vi "Taiko_Demo_WndMsg.vi"() -> ()   [LabVIEW 2010]
uses:
  Types/Taiko_Cmds.ctl
  Types/Taiko_Data.ctl
  _lib/PDLM/pdlm_lib_x86_x64_UIThread.llb/PDLM_Tag.ctl
  _lib/PDLM/pdlm_lib_x86_x64_UIThread.llb/PDLM_TaggedValue.ctl
  _lib/PDLM/pdlm_lib_x86_x64_UIThread.llb/PDLM_TaggedValueList.ctl
  <vilib>/Utility/miscctls.llb/LVRowAndColumnTypeDef.ctl
  _lib/Windows Messages for Labview/Windows messages for Labview (32 and 64).lvlib
  Types/ScaleDisplayParams.ctl
  Types/ControlAttributes.ctl
  _lib/PDLM/pdlm_lib_x86_x64_UIThread.llb/PDLM_TriggerMode.ctl
  SubVIs/AddControlsToControlStateArray.vi
  _lib/PDLM/pdlm_lib_x86_x64_UIThread.llb/PDLM_PulseTableIDs.ctl
  Types/selector.ctl
panel:
  out "Info":string="Library Version:\n1.0.64.3114\n\nSerials:\n1234567\r\n"
  in  "SetSelector":T1 caption="Select:"
  in  "LDH Pulse Table IDs":T2
  in  "Slide":sgl(slide) min=0 max=100 step=0.1 scale=0.0..100.0
  out "Tagged Value List":i32[](listbox)
  out "SystemStatus":i32(listbox)=-1
  out "SystemStatusText":string="queued error message pending\nlocked by key lock\nlocked by on/off button\nparameter changes pending\nexclusive software operation granted"
  out "QError":string="queued error message pending\nlocked by key lock\nlocked by on/off button\nparameter changes pending\nexclusive software operation granted"
  out "LH Info & Data":i32(listbox)=-1
  out "LHFeatures":i32(listbox)=-1
  out "LHFeaturesText":string="pulse mode option (int. & ext. triggerable)\ncontinuous-wave option\nburst mode option (int. triggerable)\nfan-cooled (switchable)\nintensity sensor option (type=1)"
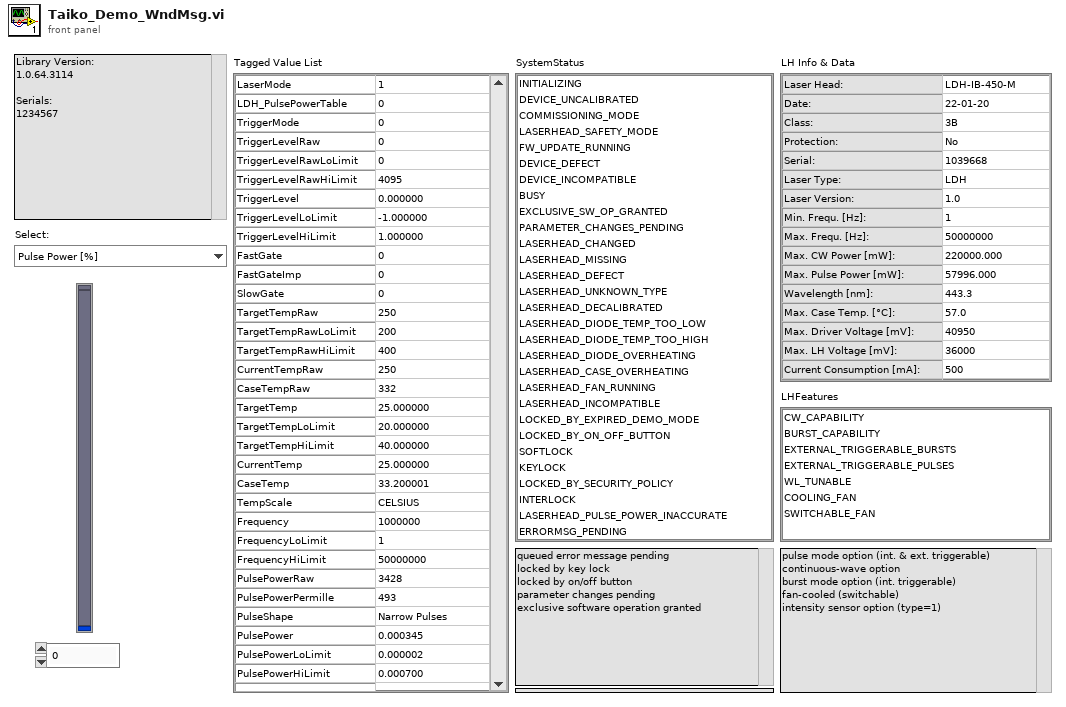
[diagram p1: front panel]
types:
  T1 = typedef "selector.ctl" = enum16{"Pulse Power [%]", "Frequency [Hz]", "Trigger Level [V]", "Pulse Table"}
  T2 = typedef "PDLM_PulseTableIDs.ctl" = enum16{"LDH_LIN_PULSE_POWER_TABLE", "LDH_MAX_PULSE_POWER_TABLE"}
  T3 = typedef "Taiko_Data.ctl" = cluster{"USBIdx":i32, "Error":errorcluster, "TaggedValueList":T4, "Ctrl State Arr":T7[], "Scale Display Params":T8}
  T4 = typedef "PDLM_TaggedValueList.ctl" = T5[]
  T5 = typedef "PDLM_TaggedValue.ctl" = cluster{"Tag":T6, "Value":u32}
  T6 = typedef "PDLM_Tag.ctl" = u32
  T7 = typedef "ControlAttributes.ctl" = cluster{"Ctl Refnum":refnum<vi>, "Visible":bool, "Enabled state":enum8{"Enabled", "Disabled", "Disabled and Grayed Out"}}
  T8 = typedef "ScaleDisplayParams.ctl" = cluster{"Style":u8, "MapMode":u8, "Increment":dbl, "Minimum":dbl, "Maximum":dbl, "Value":dbl}
  T9 = typedef "Taiko_Cmds.ctl" = enum16{"Idle", "Init", "Exit", "Update", "Error"}
  T10 = typedef "Windows messages for Labview (32 and 64).lvlib/Win Msg Queue RefNum.ctl" = refnum<k1>
  T11 = typedef "PDLM_TriggerMode.ctl" = enum32{"INTERNAL", "EXTERNAL_FALLING_EDGE", "EXTERNAL_RISING_EDGE"}
  T12 = typedef "LVRowAndColumnTypeDef.ctl" = cluster{"Row":i32, "Column":i32}
  T13 = enum16{"Pulse Power [%]", "Frequency [Hz]", "Trigger Level [V]"}
  T14 = typedef "Windows messages for Labview (32 and 64).lvlib/windows message x64.ctl" = cluster{"hWnd":u64, "Msg":u32, "wParam":u64, "lParam":i32, "time":u32, "point":cluster{"X":i32, "Y":i32}}
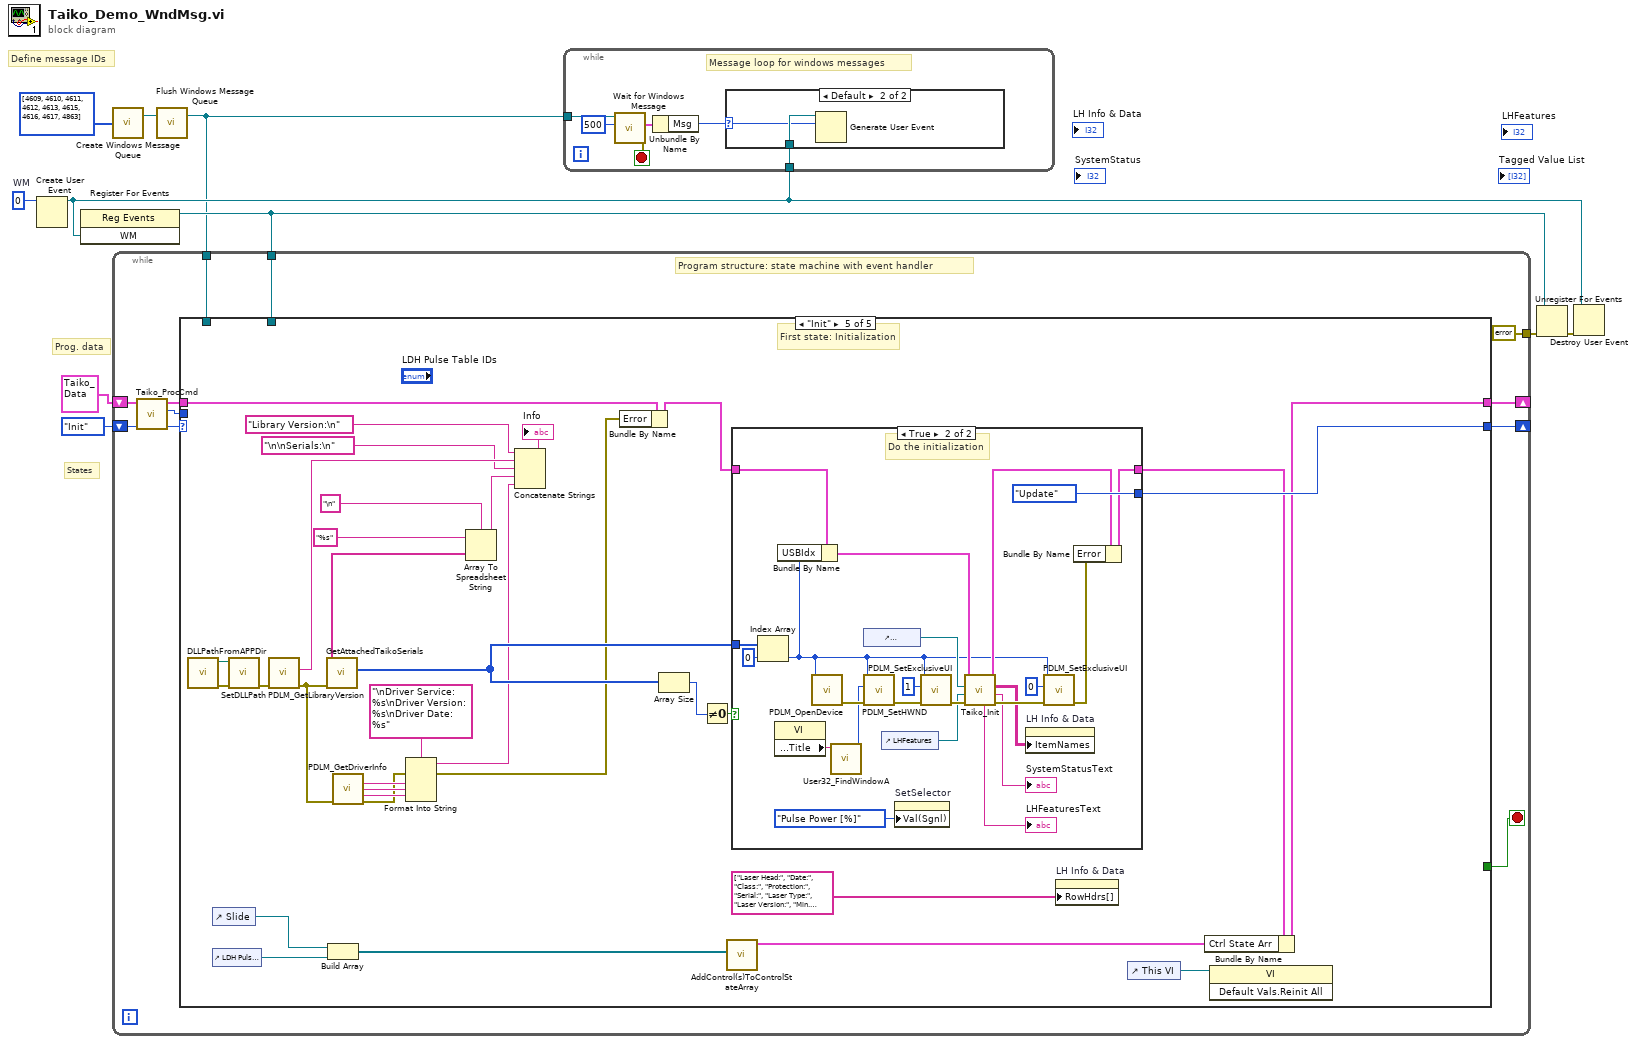
[diagram p0: block diagram]
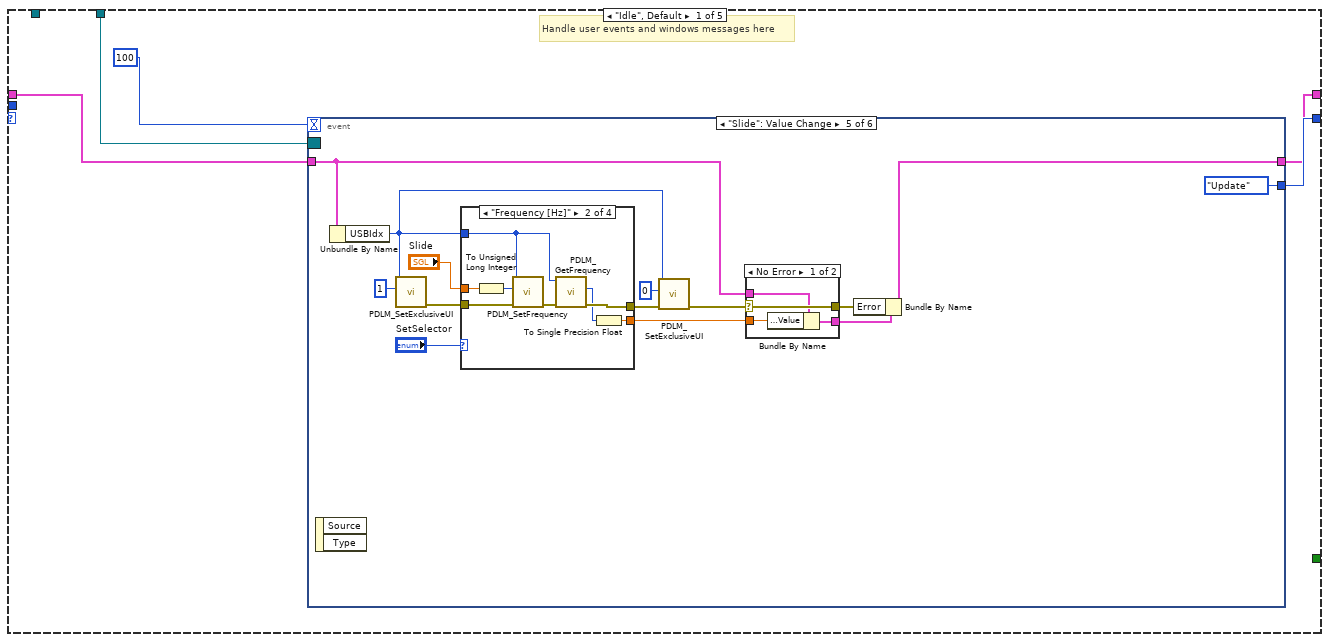
[diagram p3: hidden frame]
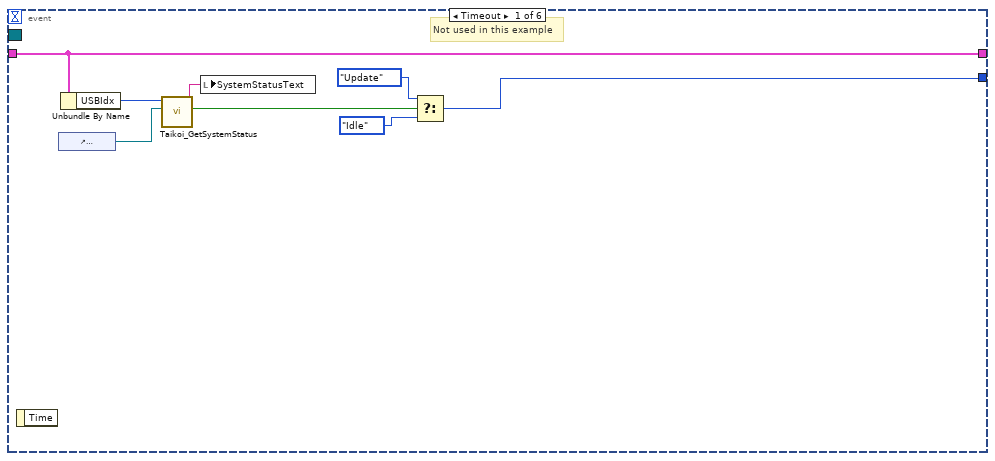
[diagram p4: hidden frame]
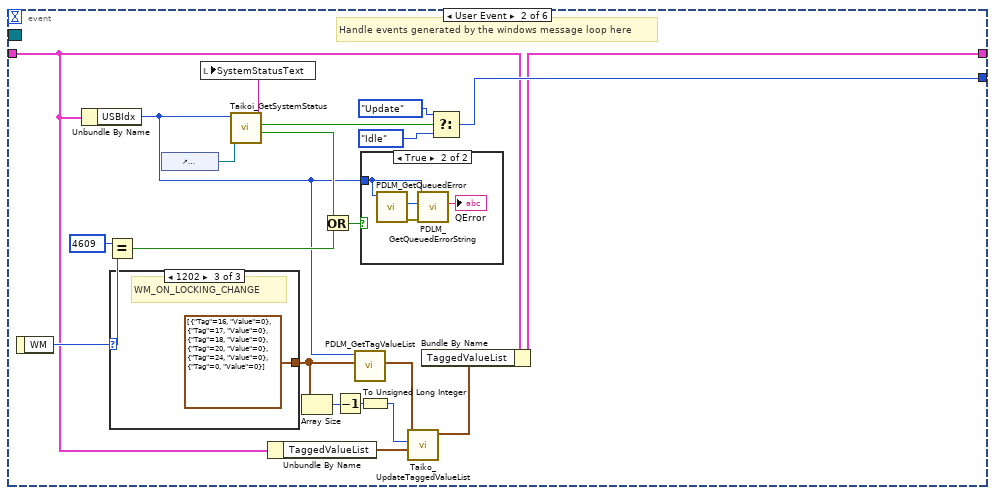
[diagram p5: hidden frame]
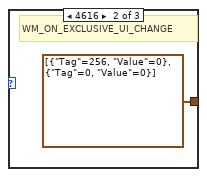
[diagram p7: hidden frame]
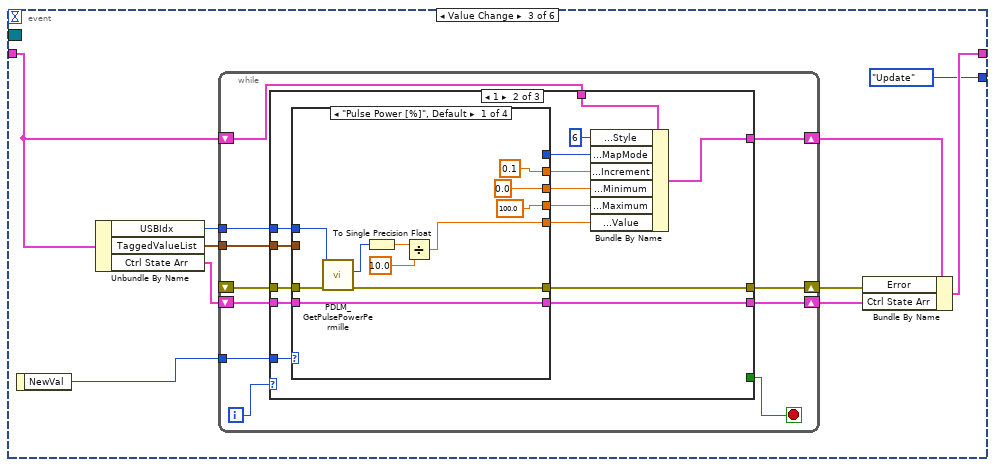
[diagram p9: hidden frame]
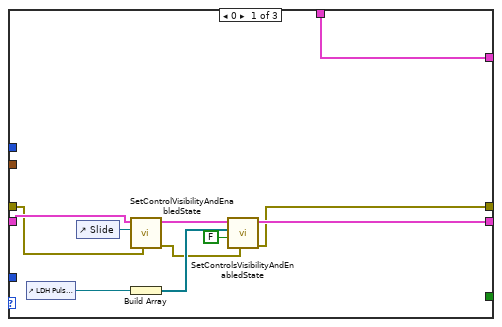
[diagram p10: hidden frame]
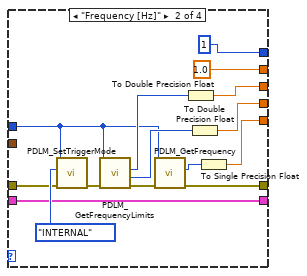
[diagram p11: hidden frame]
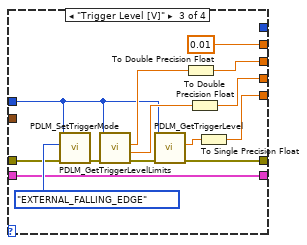
[diagram p12: hidden frame]
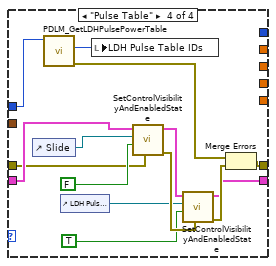
[diagram p13: hidden frame]
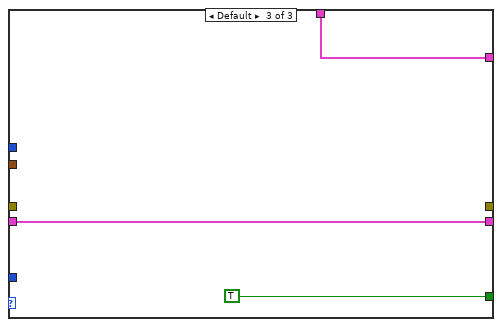
[diagram p14: hidden frame]
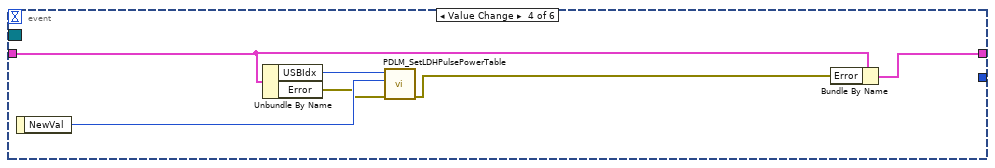
[diagram p15: hidden frame]
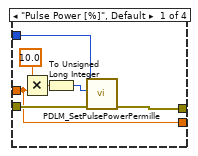
[diagram p17: hidden frame]
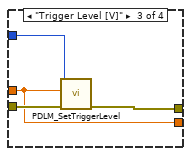
[diagram p18: hidden frame]
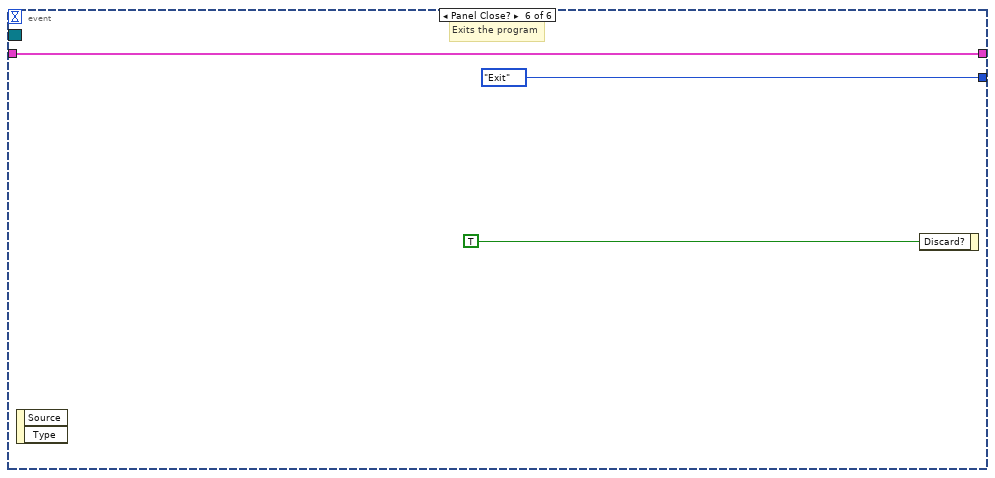
[diagram p20: hidden frame]
diagram:
  w1 = u32 0  # WM
  # "Prog. data"
  # "States"
  # "Define message IDs"
  n1 = Create User Event(user event datatype=w1) -> (user event=w3:refnum<user-event>)  [unwired: 1 in, 1 out]
  n2 = register-events(w3) -> (reference out=w6:refnum<event-registration>)  [unwired: 2 in, 1 out]
  n3 = call "Create Windows Message Queue.vi"("Messeges (none)"=u32[] [4609, 4610, 4611, 4612, 4613, 4615, 4616, 4617, 4863]) -> ("win msg queue"=w7:T10)  [unwired: 2 in, 1 out]
  n4 = call "Flush Windows Message Queue.vi"("win msg queue"=w7) -> ("win msg queue out"=w2:T10)  [unwired: 1 in, 1 out]
  n5 = while {
    shift-right: [w20] -> _
    shift-left: Taiko_Cmds."Init" ("Cmd") -> [w16]
    shift-right: [w19] -> _
    shift-left: T3 {"USBIdx"=0, "Error"={"status"=FALSE, "code"=0, "source"=""}, "TaggedValueList"=[], "Ctrl State Arr"=[], "Scale Display Params"={"Style"=0, "MapMode"=0, "Increment"=0.0, "Minimum"=0.0, "Maximum"=0.0, "Value"=0.0}} ("Data") -> [w18]
    tunnel: w6 -> [w14]
    tunnel: [errorcluster {"status"=FALSE, "code"=0, "source"=""} ("error constant")] -> w4
    tunnel: w2 -> [w12]
    stop <- w21 stop-if-true
    # "Program structure: state machine with event handler"
    n6 = call "Taiko_ProcCmd.vi"("Cmd in"=w16, "Data in"=w18) -> ("Cmd out"=w15:T9, "Cmd prev"=w11:T9, "Data out"=w17:T3)  [unwired: 7 in]
    n7 = case shown="\"Init\"" w15 {
      tunnel: [_ TRUE _ _ _] -> w21
      tunnel: [w25 _ w221 _ w296] -> w20
      tunnel: w17 -> [w23 w218 w226 w241 w295]
      tunnel: [w24 w218 w225 w249 w273] -> w19
      tunnel: w14 -> [w22 _ _ _ _]
      tunnel: w12 -> [_ w215 _ _ _]
      tunnel: w11 -> [_ _ w220 _ _]
      frame "Idle", Default {
        # "Handle user events and windows messages here"
        n8 = event shown="[4] \"Slide\": Value Change" {
          selector: w22 -> [_ _ _ _ _ _]
          dyn-events: _ -> [_ _ _ _ _ _]
          timeout: 100 -> [_ _ _ _ _ _]
          tunnel: [w29 w52 Taiko_Cmds."Update" ("Cmd") _ Taiko_Cmds."Update" ("Cmd") Taiko_Cmds."Exit" ("Cmd")] -> w25
          tunnel: [w33 w40 w63 w168 w183 w212] -> w24
          tunnel: w23 -> [w33 w41 w67 w169 w176 w212]
          event Timeout {
            # "Not used in this example"
            n9 = event-data() -> ()  [unwired: 1 in, 1 out]
            n10 = control-ref of="SystemStatus"() -> (w34:refnum<vi>)
            n11 = Unbundle By Name(w33) -> ("USBIdx"=w32:i32)
            n12 = call "Taikoi_GetSystemStatus.vi"("LBSysStatRef"=w34, "USBIdx"=w32) -> ("needUpdate"=w27:bool, "Status"=w28:string)  [unwired: 6 in, 2 out]
            n13 = local write "SystemStatusText"(w28) -> ()
            n14 = Select(t=Taiko_Cmds."Update" ("Cmd"), s=w27, f=Taiko_Cmds."Idle") -> (s? t:f=w29:T9)
          }
          event User Event {
            # "Handle events generated by the windows message loop here"
            n15 = event-data() -> ("WM"=w49:u32)  [unwired: 1 in]
            n16 = Unbundle By Name(w41) -> ("USBIdx"=w35:i32)
            n17 = Equal?(x=u32 4609, y=w49) -> (x = y?=w47:bool)
            n18 = case shown="1202" w49 {
              tunnel: [_ T4 [{"Tag"=256, "Value"=0}, {"Tag"=0, "Value"=0}] ("TaggedValueList") T4 [{"Tag"=16, "Value"=0}, {"Tag"=17, "Value"=0}, {"Tag"=18, "Value"=0}, {"Tag"=20, "Value"=0}, {"Tag"=24, "Value"=0}, {"Tag"=0, "Value"=0}] ("TaggedValueList")] -> w39
              frame 0, Default {
              }
              frame 4616 {
                # "WM_ON_EXCLUSIVE_UI_CHANGE"
              }
              frame 4610 {
                # "WM_ON_LOCKING_CHANGE"
              }
            }
            n19 = control-ref of="SystemStatus"() -> (w55:refnum<vi>)
            n20 = call "Taikoi_GetSystemStatus.vi"("LBSysStatRef"=w55, "USBIdx"=w35) -> ("QError"=w46:bool, "needUpdate"=w50:bool, "Status"=w51:string)  [unwired: 6 in, 1 out]
            n21 = local write "SystemStatusText"(w51) -> ()
            n22 = Unbundle By Name(w41) -> ("TaggedValueList"=w42:T4)
            n23 = Array Size(array=w39) -> (size(s)=w38:i32)
            n24 = Or(x=w46, y=w47) -> (x .or. y?=w45:bool)
            n25 = Decrement(x=w38) -> (x-1=w37:i32)
            n26 = call "PDLM_GetTagValueList.vi"("TaggedValueList"=w39, "USBIdx"=w35) -> ("TaggedValueList out"=w44:T4)  [unwired: 7 in, 2 out]
            n27 = To Unsigned Long Integer(number=w37) -> (unsigned 32bit integer=w36:u32)
            n28 = case shown="True" w45 {
              tunnel: w35 -> [_ w59]
              frame False {
              }
              frame True {
                n29 = call "PDLM_GetQueuedError.vi"("USBIdx"=w59) -> ("error out"=w61:errorcluster, "ErrCode"=w60:i32)  [unwired: 8 in, 1 out]
                n30 = call "PDLM_GetQueuedErrorString.vi"("error in (no error)"=w61, "ErrCode"=w60, "USBIdx"=w59) -> ("ErrText"=→"QError":string)  [unwired: 6 in, 2 out]
              }
            }
            n31 = call "Taiko_UpdateTaggedValueList.vi"("TaggedValueList all"=w42, "ListLen in"=w36, "TaggedValueList in"=w44) -> ("TaggedValueList"=w43:T4)  [unwired: 7 in, 1 out]
            n32 = Bundle By Name(cluster=w41, "TaggedValueList"=w43) -> (w40:T3)
            n33 = Select(t=Taiko_Cmds."Update" ("Cmd"), s=w50, f=Taiko_Cmds."Idle") -> (s? t:f=w52:T9)
          }
          event Value Change {
            n34 = event-data() -> ("NewVal"=w68:T1)  [unwired: 1 in]
            n35 = Unbundle By Name(w67) -> ("USBIdx"=w69:i32, "TaggedValueList"=w70:T4, "Ctrl State Arr"=w71:T7[])
            n36 = while {
              tunnel: w69 -> [w82]
              tunnel: w68 -> [w81]
              tunnel: w70 -> [w79]
              shift-right: [w78] -> w66
              shift-left: w71 -> [w77]
              shift-right: [w80] -> w65
              shift-left: _ -> [w74]
              shift-right: [w72] -> w64
              shift-left: w67 -> [w73]
              i -> [w76]
              stop <- w75 stop-if-true
              n37 = case shown="1" w76 {
                tunnel: w82 -> [_ w108 _]
                tunnel: w81 -> [_ w107 _]
                tunnel: [w84 w106 _] -> w80
                tunnel: w79 -> [_ w105 _]
                tunnel: [w88 w103 w164] -> w78
                tunnel: w77 -> [w90 w104 w164]
                tunnel: [_ _ TRUE] -> w75
                tunnel: w74 -> [w83 w102 _]
                tunnel: w73 -> [w87 w101 w163]
                tunnel: [w87 w100 w163] -> w72
                frame 0 {
                  n38 = control-ref of="LDH Pulse Table IDs"() -> (w86:refnum<vi>)
                  n39 = control-ref of="Slide"() -> (w92:refnum<vi>)
                  n40 = call "SetControlVisibilityAndEnabledState.vi"("error in (no error)"=w83, "Ctl Refnum"=w92, "Control State Array"=w90) -> ("error out"=w85:errorcluster, "Control State Array (out)"=w91:T7[])  [unwired: 7 in]
                  n41 = Build Array(w86) -> (w93:refnum<vi>[])
                  n42 = call "SetControlsVisibilityAndEnabledState.vi"("error in (no error)"=w85, "Visible (T)"=FALSE, "Array"=w93, "Control State Array"=w91) -> ("error out"=w84:errorcluster, "Control State Array (out)"=w88:T7[])  [unwired: 6 in]
                }
                frame 1 {
                  n43 = case shown="\"Pulse Power [%]\", Default" w107 {
                    tunnel: w108 -> [w116 w123 w138 w153]
                    tunnel: [0.0 w131 w146 _] -> w96
                    tunnel: [100.0 w129 w144 _] -> w95
                    tunnel: [w112 w127 w143 _] -> w94
                    tunnel: [w115 w133 w147 w152] -> w106
                    tunnel: [0.1 ("Data Entry Limits:Increment") 1.0 ("Data Entry Limits:Increment") 0.01 ("Data Entry Limits:Increment") _] -> w97
                    tunnel: [_ u8 1 ("Scale.Mapping Mode") _ _] -> w98
                    tunnel: w105 -> [_ _ _ _]
                    tunnel: w104 -> [w110 w121 w136 w160]
                    tunnel: [w110 w121 w136 w155] -> w103
                    tunnel: w102 -> [w109 w120 w135 w159]
                    frame "Pulse Power [%]", Default {
                      n44 = call "PDLM_GetPulsePowerPermille.vi"("error in (no error)"=w109, "USBIdx"=w116) -> ("error out"=w115:errorcluster, "permille"=w114:u32)  [unwired: 7 in, 1 out]
                      n45 = To Single Precision Float(number=w114) -> (single precision float=w113:sgl)
                      n46 = Divide(x=w113, y=sgl 10.0) -> (x/y=w112:sgl)
                    }
                    frame "Frequency [Hz]" {
                      n47 = call "PDLM_SetTriggerMode.vi"("error in (no error)"=w120, "mode"=PDLM_TriggerMode."INTERNAL", "USBIdx"=w123) -> ("error out"=w124:errorcluster)  [unwired: 7 in, 1 out]
                      n48 = call "PDLM_GetFrequencyLimits.vi"("error in (no error)"=w124, "USBIdx"=w123) -> ("error out"=w134:errorcluster, "MaxFreq"=w130:u32, "MinFreq"=w132:u32)  [unwired: 6 in, 1 out]
                      n49 = call "PDLM_GetFrequency.vi"("error in (no error)"=w134, "USBIdx"=w123) -> ("error out"=w133:errorcluster, "freq"=w128:u32)  [unwired: 7 in, 1 out]
                      n50 = To Double Precision Float(number=w132) -> (double precision float=w131:dbl)
                      n51 = To Double Precision Float(number=w130) -> (double precision float=w129:dbl)
                      n52 = To Single Precision Float(number=w128) -> (single precision float=w127:sgl)
                    }
                    frame "Trigger Level [V]" {
                      n53 = call "PDLM_SetTriggerMode.vi"("error in (no error)"=w135, "mode"=PDLM_TriggerMode."EXTERNAL_FALLING_EDGE", "USBIdx"=w138) -> ("error out"=w139:errorcluster)  [unwired: 7 in, 1 out]
                      n54 = call "PDLM_GetTriggerLevelLimits.vi"("error in (no error)"=w139, "USBIdx"=w138) -> ("error out"=w148:errorcluster, "MaxLevel"=w145:sgl, "MinLevel"=w141:sgl)  [unwired: 6 in, 1 out]
                      n55 = call "PDLM_GetTriggerLevel.vi"("error in (no error)"=w148, "USBIdx"=w138) -> ("error out"=w147:errorcluster, "Level"=w140:sgl)  [unwired: 7 in, 1 out]
                      n56 = To Double Precision Float(number=w141) -> (double precision float=w146:dbl)
                      n57 = To Double Precision Float(number=w145) -> (double precision float=w144:dbl)
                      n58 = To Single Precision Float(number=w140) -> (single precision float=w143:sgl)
                    }
                    frame "Pulse Table" {
                      n59 = control-ref of="Slide"() -> (w149:refnum<vi>)
                      n60 = call "PDLM_GetLDHPulsePowerTable.vi"("USBIdx"=w153) -> ("error out"=w151:errorcluster, "TableIdx (out)"=w154:u32)  [unwired: 8 in, 1 out]
                      n61 = control-ref of="LDH Pulse Table IDs"() -> (w150:refnum<vi>)
                      n62 = local write "LDH Pulse Table IDs"(w154) -> ()
                      n63 = call "SetControlVisibilityAndEnabledState.vi"("error in (no error)"=w159, "Visible (T)"=FALSE, "Ctl Refnum"=w149, "Control State Array"=w160) -> ("error out"=w158:errorcluster, "Control State Array (out)"=w162:T7[])  [unwired: 6 in]
                      n64 = call "SetControlVisibilityAndEnabledState.vi"("error in (no error)"=w158, "Visible (T)"=TRUE, "Ctl Refnum"=w150, "Control State Array"=w162) -> ("error out"=w157:errorcluster, "Control State Array (out)"=w155:T7[])  [unwired: 6 in]
                      n65 = Merge Errors(w151, w157) -> (w152:errorcluster)
                    }
                  }
                  n66 = Bundle By Name(cluster=w101, "Scale Display Params.Style"=u8 6, "Scale Display Params.MapMode"=w98, "Scale Display Params.Increment"=w97, "Scale Display Params.Minimum"=w96, "Scale Display Params.Maximum"=w95, "Scale Display Params.Value"=w94) -> (w100:T3)
                }
                frame Default {
                }
              }
            }
            n67 = Bundle By Name(cluster=w64, "Error"=w65, "Ctrl State Arr"=w66) -> (w63:T3)
          }
          event Value Change {
            n68 = event-data() -> ("NewVal"=w167:T2)  [unwired: 1 in]
            n69 = Unbundle By Name(w169) -> ("USBIdx"=w171:i32, "Error"=w166:errorcluster)
            n70 = call "PDLM_SetLDHPulsePowerTable.vi"("error in (no error)"=w166, "TableIdx"=w167, "USBIdx"=w171) -> ("error out"=w170:errorcluster)  [unwired: 7 in, 1 out]
            n71 = Bundle By Name(cluster=w169, "Error"=w170) -> (w168:T3)
          }
          event "Slide": Value Change {
            n72 = event-data() -> ()  [unwired: 1 in, 2 out]
            n73 = Unbundle By Name(w176) -> ("USBIdx"=w178:i32)
            n74 = call "PDLM_SetExclusiveUI.vi"("mode"=u32 1, "USBIdx"=w178) -> ("error out"=w182:errorcluster)  [unwired: 8 in, 1 out]
            n75 = case shown="\"Frequency [Hz]\"" "SetSelector" {
              tunnel: w178 -> [w198 w203 w210 _]
              tunnel: "Slide" -> [w192 w204 w207 _]
              tunnel: [w193 w201 w208 w211] -> w179
              tunnel: w182 -> [w197 w205 w209 w211]
              tunnel: [w192 w199 w207 _] -> w173
              frame "Pulse Power [%]", Default {
                n76 = Multiply(x=sgl 10.0, y=w192) -> (x*y=w195:sgl)
                n77 = To Unsigned Long Integer(number=w195) -> (unsigned 32bit integer=w194:u32)
                n78 = call "PDLM_SetPulsePowerPermille.vi"("error in (no error)"=w197, "permille"=w194, "USBIdx"=w198) -> ("error out"=w193:errorcluster)  [unwired: 7 in, 1 out]
              }
              frame "Frequency [Hz]" {
                n79 = To Unsigned Long Integer(number=w204) -> (unsigned 32bit integer=w206:u32)
                n80 = call "PDLM_SetFrequency.vi"("error in (no error)"=w205, "freq"=w206, "USBIdx"=w203) -> ("error out"=w202:errorcluster)  [unwired: 7 in, 1 out]
                n81 = call "PDLM_GetFrequency.vi"("error in (no error)"=w202, "USBIdx"=w203) -> ("error out"=w201:errorcluster, "freq"=w200:u32)  [unwired: 7 in, 1 out]
                n82 = To Single Precision Float(number=w200) -> (single precision float=w199:sgl)
              }
              frame "Trigger Level [V]" {
                n83 = call "PDLM_SetTriggerLevel.vi"("error in (no error)"=w209, "Level"=w207, "USBIdx"=w210) -> ("error out"=w208:errorcluster)  [unwired: 7 in, 1 out]
              }
              frame "Pulse Table" {
              }
            }
            n84 = call "PDLM_SetExclusiveUI.vi"("error in (no error)"=w179, "mode"=u32 0, "USBIdx"=w178) -> ("error out"=w177:errorcluster)  [unwired: 7 in, 1 out]
            n85 = case shown="No Error" w177 {
              selector: w177 -> [w189 w190]
              tunnel: [w189 w190] -> w174
              tunnel: w176 -> [w188 w191]
              tunnel: [w187 w191] -> w175
              tunnel: w173 -> [w186 _]
              frame No Error {
                n86 = Bundle By Name(cluster=w188, "Scale Display Params.Value"=w186) -> (w187:T3)
              }
              frame Error {
              }
            }
            n87 = Bundle By Name(cluster=w175, "Error"=w174) -> (w183:T3)
          }
          event Panel Close? {
            # "Exits the program"
            n88 = event-data() -> ()  [unwired: 1 in, 2 out]
            n89 = event-data("Discard?"=TRUE) -> ()  [unwired: 1 in, 1 out]
          }
        }
      }
      frame "Exit" {
        # "Close the device and release the message queue"
        n90 = call "Destroy Windows Message Queue.vi"("win msg queue"=w215) -> ()  [unwired: 1 in, 1 out]
        n91 = Unbundle By Name(w218) -> ("USBIdx"=w217:i32)
        n92 = call "PDLM_CloseDevice.vi"("USBIdx"=w217) -> ()  [unwired: 9 in, 2 out]
      }
      frame "Error" {
        # "Handle errors here (adapt to your own needs, e.g. define exception list etc.)"
        n93 = Unbundle By Name(w226) -> ("Error"=w219:errorcluster)
        n94 = call "Taiko_ErrorDlg.vi"("Error in"=w219) -> ("Exit"=w223:bool)  [unwired: 9 in, 1 out]
        n95 = Bundle By Name(cluster=w226, "Error"=errorcluster {"status"=FALSE, "code"=0, "source"=""}) -> (w225:T3)
        n96 = Select(t=Taiko_Cmds."Exit" ("Cmd"), s=w223, f=w220) -> (s? t:f=w221:T9)
      }
      frame "Update" {
        # "Get all pending changes here and update controls"
        n97 = Unbundle By Name(w241) -> ("USBIdx"=w240:i32, "TaggedValueList"=w246:T4, "Ctrl State Arr"=w229:T7[], "Scale Display Params"=w230:T8)
        n98 = call "GetEmptyTagValueList.vi"() -> ("Array"=w231:T5[])  [unwired: 10 in, 1 out]
        n99 = Unbundle(w230) -> ("Style"=w238:u8, "MapMode"=w237:u8, "Increment"=w236:dbl, "Minimum"=w235:dbl, "Maximum"=w234:dbl, "Value"=w233:dbl)
        n100 = call "PDLM_GetQueuedChanges.vi"("TaggedValueList"=w231, "USBIdx"=w240) -> ("error out"=w228:errorcluster, "ListLen out"=w248:u32, "TaggedValueList out"=w247:T4)  [unwired: 6 in, 1 out]
        n101 = call "SetControlsEnableDisableVisibleStates.vi"("Array"=w229) -> ("error out"=w239:errorcluster)  [unwired: 10 in]
        n102 = property on="Slide" class="Slide (strict)"("Scale.Style"=w238, "Scale.Mapping Mode"=w237, "Increment"=w236, "Scale.Increment"=w236, "Minimum"=w235, "Scale.Minimum"=w235, "Maximum"=w234, "Scale.Maximum"=w234, "Value"=w233) -> (error out=w232:errorcluster)  [unwired: 2 in, 1 out]
        n103 = Merge Errors(w228, w239, w232) -> (w227:errorcluster)
        n104 = call "Taiko_UpdateTaggedValueList.vi"("TaggedValueList all"=w246, "ListLen in"=w248, "TaggedValueList in"=w247) -> ("Array"=w244:i32[], "TaggedValueList"=w245:T4)  [unwired: 7 in]
        n105 = Array Size(array=w244) -> (size(s)=w243:i32)
        n106 = Not Equal To 0?(x=w243) -> (x != 0?=w242:bool)
        n107 = case shown="True" w242 {
          tunnel: w245 -> [_ w255]
          tunnel: w244 -> [_ w250]
          tunnel: w241 -> [_ _]
          frame False {
          }
          frame True {
            n108 = call "Taiko_TaggedValueListToStrArray.vi"("TaggedValueList"=w255) -> ("ValList"=w256:string[], "TagList"=w258:string[])  [unwired: 9 in]
            n109 = Build Array(w256) -> (w257:string[][])
            n110 = Transpose 2D Array(2D array=w257) -> (transposed array=w259:string[][])
            n111 = property on="Tagged Value List" class="MCListbox (strict)"("ActiveCell"=T12 {"Row"=-2, "Column"=-2} ("Active Cell:Active Cell"), "CellBG"=u32 16777215, "CellFontColor"=u32 0, "RowHdrs[]"=w258, "ItemNames"=w259) -> (error out=w251:errorcluster)  [unwired: 2 in, 1 out]
            n112 = for {
              tunnel: w250 -> [w264] mode=indexing
              tunnel: w251 -> [w260]
              n113 = Bundle By Name(cluster=T12 {"Row"=0, "Column"=0} ("Active Cell:Active Cell"), "Row"=w264) -> (w263:T12)
              n114 = property on="Tagged Value List" class="MCListbox (strict)"(error in=w260, "ActiveCell"=w263, "CellBG"=u32 255 ("Color Box"), "CellFontColor"=u32 16777215) -> ()  [unwired: 1 in, 2 out]
            }
          }
        }
        n115 = Bundle By Name(cluster=w241, "Error"=w227, "TaggedValueList"=w245) -> (w249:T3)
      }
      frame "Init" {
        # "First state: Initialization"
        n116 = call "DLLPathFromAPPDir.vi"() -> ("error out"=w267:errorcluster, "DLLPath"=w268:path)  [unwired: 10 in]
        n117 = control-ref of="Slide"() -> (w276:refnum<vi>)
        n118 = control-ref of="LDH Pulse Table IDs"() -> (w275:refnum<vi>)
        n119 = call "SetDLLPath.vi"("error in (no error)"=w267, "DLLPath"=w268) -> ("error out"=w266:errorcluster)  [unwired: 9 in]
        n120 = call "PDLM_GetLibraryVersion.vi"("error in (no error)"=w266) -> ("error out"=w278:errorcluster, "Version"=w291:string)  [unwired: 8 in, 1 out]
        n121 = call "GetAttachedTaikoSerials.vi"("error in (no error)"=w278) -> ("Array 2"=w284:i32[], "Array"=w285:string[])  [unwired: 9 in]
        n122 = Build Array(w276, w275) -> (w274:refnum<vi>[])
        n123 = call "PDLM_GetDriverInfo.vi"("error in (no error)"=w278) -> ("cName"=w282:string, "cVersion"=w281:string, "cDate"=w280:string, "error out"=w279:errorcluster)  [unwired: 10 in, 1 out]
        n124 = Format Into String(format string="\nDriver Service: %s\nDriver Version: %s\nDriver Date: %s" ("string"), error in=w279, w282, w281, w280) -> (resulting string=w277:string, error out=w269:errorcluster)  [unwired: 1 in]
        n125 = Array To Spreadsheet String(delimiter (Tab)="\n", array=w285, 3:"%s" ("format string")) -> (spreadsheet string=w290:string)
        n126 = Concatenate Strings("Library Version:\n" ("string"), w291, "\n\nSerials:\n" ("string"), w290, w277) -> (→"Info":string)
        n127 = Bundle By Name(cluster=w295, "Error"=w269) -> (w270:T3)
        n128 = Array Size(array=w284) -> (size(s)=w298:i32)
        n129 = Not Equal To 0?(x=w298) -> (x != 0?=w297:bool)
        n130 = call-poly "AddControl(s)ToControlStateArray.vi"("Array"=w274) -> ("Control State Array (out)"=w272:T7[])  [unwired: 9 in, 1 out]
        n131 = case shown="True" w297 {
          tunnel: w284 -> [_ w322]
          tunnel: [Taiko_Cmds."Exit" ("Cmd") Taiko_Cmds."Update" ("Cmd")] -> w296
          tunnel: w270 -> [w299 w311]
          tunnel: [w299 w318] -> w294
          frame False {
            # "No device to open found"
          }
          frame True {
            # "Do the initialization"
            n132 = Index Array(array=w322, index=0) -> (element=w304:i32)
            n133 = property class="VI"() -> ("Front Panel.Title"=w302:string)  [unwired: 2 in, 2 out]
            n134 = Bundle By Name(cluster=w311, "USBIdx"=w304) -> (w310:T3)
            n135 = call "PDLM_OpenDevice.vi"("USBIdx"=w304) -> ("error out"=w306:errorcluster)  [unwired: 8 in, 2 out]
            n136 = call "User32_FindWindowA.vi"("lpszWindowName"=w302) -> ("hWnd"=w303:u64)  [unwired: 9 in, 1 out]
            n137 = control-ref of="SystemStatus"() -> (w313:refnum<vi>)
            n138 = call "PDLM_SetHWND.vi"("error in (no error)"=w306, "hwnd"=w303, "USBIdx"=w304) -> ("error out"=w305:errorcluster)  [unwired: 7 in, 1 out]
            n139 = control-ref of="LHFeatures"() -> (w312:refnum<vi>)
            n140 = property on="SetSelector" class="Enum (strict)"("Val(Sgnl)"=T13."Pulse Power [%]" ("Value (Signaling)")) -> ()  [unwired: 2 in, 2 out]
            n141 = call "PDLM_SetExclusiveUI.vi"("error in (no error)"=w305, "mode"=u32 1, "USBIdx"=w304) -> ("error out"=w316:errorcluster)  [unwired: 7 in, 1 out]
            n142 = call "Taiko_Init.vi"("error in (no error)"=w316, "LBLHFeaturesRef"=w312, "LBSysStatRef"=w313, "Data"=w310) -> ("error out"=w315:errorcluster, "Status"=→"SystemStatusText":string, "LHInfoData"=w309:string[][], "Data out"=w307:T3, "Features"=→"LHFeaturesText":string)  [unwired: 3 in]
            n143 = property on="LH Info & Data" class="MCListbox (strict)"("ItemNames"=w309) -> ()  [unwired: 2 in, 2 out]
            n144 = call "PDLM_SetExclusiveUI.vi"("error in (no error)"=w315, "mode"=u32 0, "USBIdx"=w304) -> ("error out"=w317:errorcluster)  [unwired: 7 in, 1 out]
            n145 = Bundle By Name(cluster=w307, "Error"=w317) -> (w318:T3)
          }
        }
        n146 = property on="LH Info & Data" class="MCListbox (strict)"("RowHdrs[]"=string[] ["Laser Head:", "Date:", "Class:", "Protection:", "Serial:", "Laser Type:", "Laser Version:", "Min. Frequ. [Hz]:", "Max. Frequ. [Hz]:", "Max. CW Power [mW]:", "Max. Pulse Power [mW]:", "Wavelength [nm]:", "Max. Case Temp. [°C]:", "Max. Driver Voltage [mV]:", "Max. LH Voltage [mV]:", "Current Consumption [mA]:", "Calib. Warranty [h]:"] ("Row Header Strings[]")) -> ()  [unwired: 2 in, 2 out]
        n147 = control-ref of="This VI"() -> (w271:refnum<vi>)
        n148 = Bundle By Name(cluster=w294, "Ctrl State Arr"=w272) -> (w273:T3)
        n149 = invoke class="VI" method="Default Vals.Reinit All"(reference=w271) -> ()  [unwired: 2 in, 3 out]
      }
    }
  }
  n150 = while {
    tunnel: w2 -> [w329]
    tunnel: w3 -> [w327]
    stop <- w326 stop-if-true
    # "Message loop for windows messages"
    n151 = call "Wait for Windows Message.vi"("win msg queue"=w329, "ms timeout (-1)"=500) -> ("Message"=w328:T14, "error out"=w326:errorcluster)  [unwired: 2 in, 4 out]
    n152 = Unbundle By Name(w328) -> ("Msg"=w324:u32)
    n153 = case shown="Default" w324 {
      selector: w324 -> [_ w330]
      tunnel: w327 -> [_ w331]
      frame 0 {
      }
      frame Default {
        # "WM_ON_PARAMETER_CHANGE"
        n154 = Generate User Event(user event=w331, event data cluster=w330) -> ()  [unwired: 1 in, 2 out]
      }
    }
  }
  n155 = Unregister For Events(event registration refnum=w6, error in=w4) -> (error out=w5:errorcluster)
  n156 = Destroy User Event(user event=w3, error in=w5) -> ()  [unwired: 1 out]
